vi "catalan1.vi"(10 "n":i32) -> (2 "ans":i32)   [LabVIEW 2023]
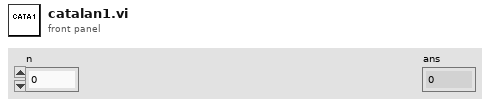
[diagram p1: front panel]
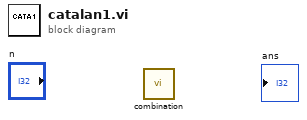
[diagram p0: block diagram]
diagram:
  n1 = call "combination.vi"() -> ()  [unwired: 11 in, 1 out]
